vi "COB send.vi"(4 "Data":u8[](array[numeric]), 5 "error in (no error)":errorcluster, 7 "COB id":i32, 8 "Handle in":i32) -> (0 "error out":errorcluster, 3 "Handle out":i32)   [LabVIEW 2017, in "canopen.lvlib" / "CANopen.lvclass"]
doc: "Sends a bunch of data to a specific COB-ID."
uses:
  CANopen.lvclass
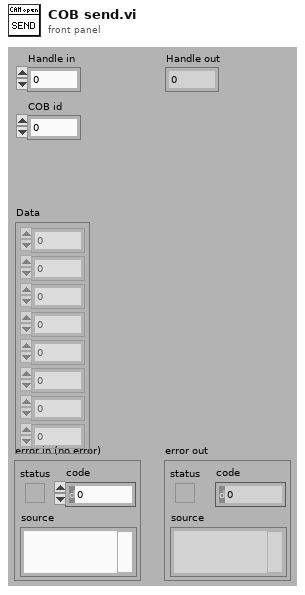
[diagram p1: front panel]
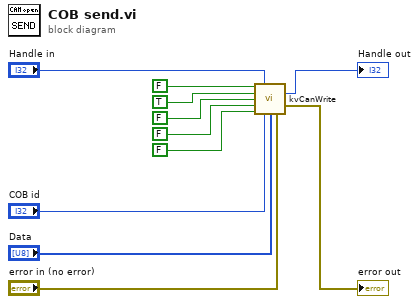
[diagram p0: block diagram]
diagram:
  n1 = call <userlib>:"kvCanWrite.vi"("Remote Request"=FALSE, "Channel Handle (input only)"="Handle in", "error in (no error)"="error in (no error)", "Standard 11-bit Id"=TRUE, "Extended 29-bit Id"=FALSE, "Error Frame"=FALSE, "Wakeup"=FALSE, "Message Id"="COB id", "Message"="Data") -> ("Channel Handle (output only)"=→"Handle out":i32, "error out"=→"error out":errorcluster)  [unwired: 5 out]
